vi "Report.vi"() -> ()   [LabVIEW 2019]
uses:
  <vilib>/Utility/NIReport.llb/Report Type.ctl
  <vilib>/addons/_office/excel.llb/Excel Get Data ([str]).vi
  <vilib>/Utility/NIReport.llb/Append Text Table to Report (wrap).vi
  <vilib>/Utility/NIReport.llb/NI_report.lvclass
  <vilib>/Utility/NIReport.llb/NI_ReportGenerationCore.lvlib
  <vilib>/addons/_office/NI_ReportGenerationToolkit.lvlib
  <vilib>/Utility/NIReport.llb/Excel/NI_Excel.lvclass
panel:
  out "data 5":string[][](array[string])
  out "data 4":string[][](array[string])
  out "data 3":string[][](array[string])
  out "data":string[][](array[string])
  out "data 2":string[][](array[string])
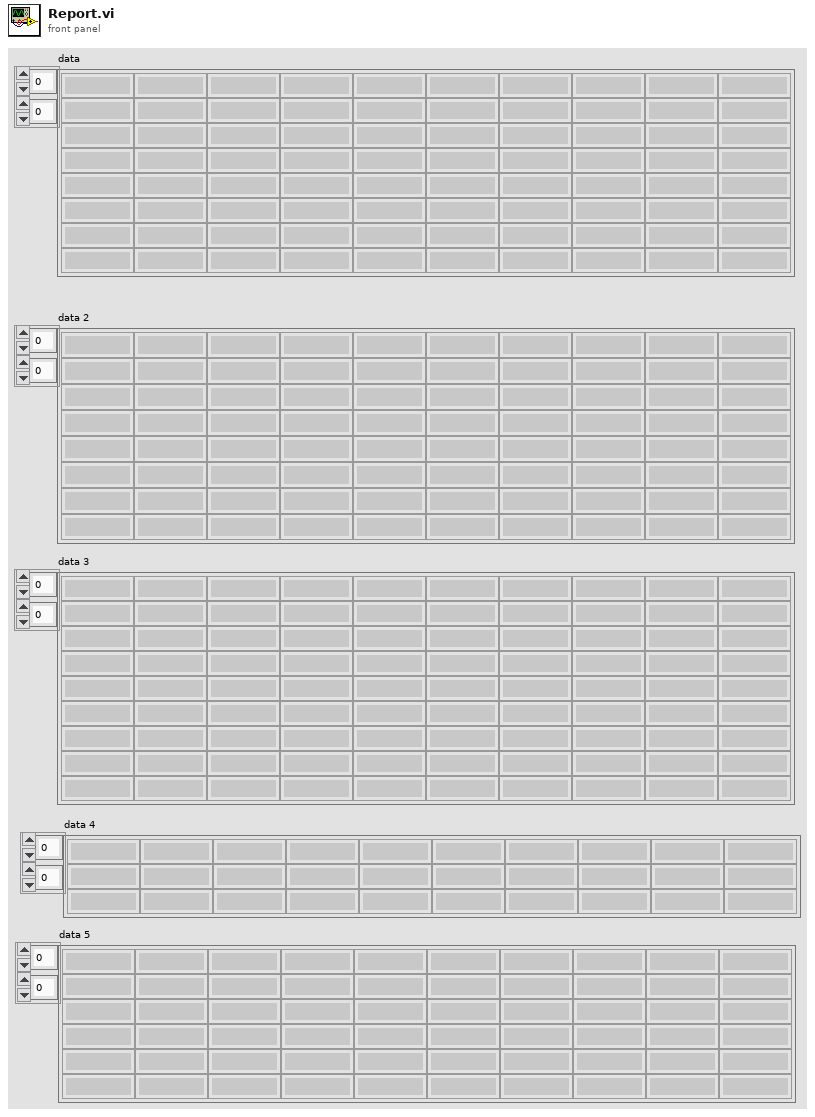
[diagram p1: front panel]
types:
  T1 = typedef "NI_ReportGenerationCore.lvlib/Report Type.ctl" = enum16{"HTML", "Word", "Excel"}
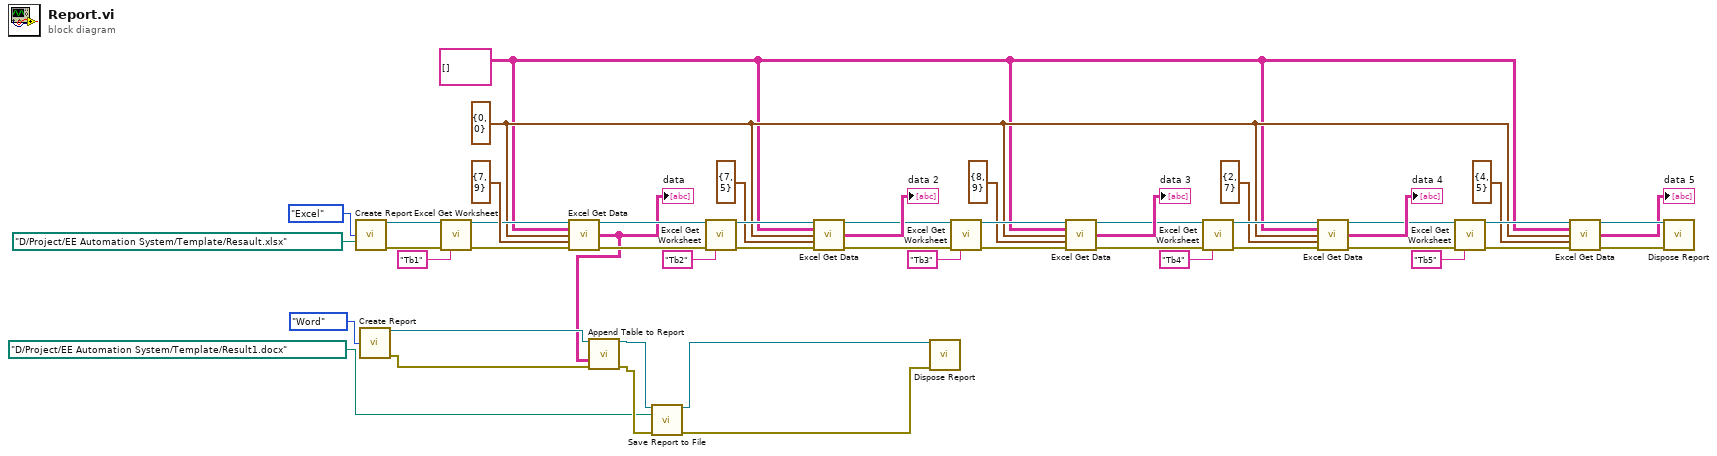
[diagram p0: block diagram]
diagram:
  w7 = string[][] [] ("data type")
  w15 = cluster{"row":i32, "column":i32} {"row"=0, "column"=0} ("start (-1, -1)")
  n1 = call <vilib>:"Create Report.vi"("report type"=Report_Type."Excel", "template (empty)"=path "D:/Project/EE Automation System/Template/Resault.xlsx") -> ("report out"=w43:refnum<class "NI_report.lvclass">, "error out"=w39:errorcluster)  [unwired: 12 in]
  n2 = call <vilib>:"Create Report.vi"("report type"=Report_Type."Word") -> ("report out"=w9:refnum<class "NI_report.lvclass">, "error out"=w8:errorcluster)  [unwired: 13 in]
  n3 = call <vilib>:"Excel Get Worksheet.vi"("report in"=w43, "error in (no error)"=w39, "name (\"\")"="Tb1" ("name (\"\")")) -> ("report out"=w45:refnum<class "NI_report.lvclass">, "error out"=w44:errorcluster)  [unwired: 11 in]
  n4 = call-poly <vilib>:"Excel Get Data.vi"("report in"=w45, "data type"=w7, "start (-1, -1)"=w15, "end (-1, -1)"=cluster{"row":i32, "column":i32} {"row"=7, "column"=9}, "error in (no error)"=w44) -> ("report out"=w36:refnum<class "NI_report.lvclass">, "data"=w1:string[][], "error out"=w35:errorcluster)  [unwired: 8 in]
  "data" <- w1
  n5 = call-poly <vilib>:"Append Table to Report.vi"("report in"=w9, "text data"=w1, "error in (no error)"=w8) -> ("report out"=w6:refnum<class "NI_report.lvclass">, "error out"=w5:errorcluster)  [unwired: 9 in, 2 out]
  n6 = call-dynamic "Save Report to File.vi"("report in"=w6, "report file path"=path "D:/Project/EE Automation System/Template/Result1.docx" ("template (empty)"), "error in (no error)"=w5) -> ("report out"=w3:refnum<class "NI_report.lvclass">, "error out"=w4:errorcluster)  [unwired: 11 in]
  n7 = call <vilib>:"Excel Get Worksheet.vi"("report in"=w36, "error in (no error)"=w35, "name (\"\")"="Tb2" ("name (\"\")")) -> ("report out"=w41:refnum<class "NI_report.lvclass">, "error out"=w40:errorcluster)  [unwired: 11 in]
  n8 = call-poly <vilib>:"Excel Get Data.vi"("report in"=w41, "data type"=w7, "start (-1, -1)"=w15, "end (-1, -1)"=cluster{"row":i32, "column":i32} {"row"=7, "column"=5}, "error in (no error)"=w40) -> ("report out"=w33:refnum<class "NI_report.lvclass">, "data"=→"data 2":string[][], "error out"=w34:errorcluster)  [unwired: 8 in]
  n9 = call-dynamic "Dispose Report.vi"("report in"=w3, "error in (no error)"=w4) -> ()  [unwired: 13 in, 1 out]
  n10 = call <vilib>:"Excel Get Worksheet.vi"("report in"=w33, "error in (no error)"=w34, "name (\"\")"="Tb3" ("name (\"\")")) -> ("report out"=w31:refnum<class "NI_report.lvclass">, "error out"=w30:errorcluster)  [unwired: 11 in]
  n11 = call-poly <vilib>:"Excel Get Data.vi"("report in"=w31, "data type"=w7, "start (-1, -1)"=w15, "end (-1, -1)"=cluster{"row":i32, "column":i32} {"row"=8, "column"=9}, "error in (no error)"=w30) -> ("report out"=w26:refnum<class "NI_report.lvclass">, "data"=→"data 3":string[][], "error out"=w27:errorcluster)  [unwired: 8 in]
  n12 = call <vilib>:"Excel Get Worksheet.vi"("report in"=w26, "error in (no error)"=w27, "name (\"\")"="Tb4" ("name (\"\")")) -> ("report out"=w23:refnum<class "NI_report.lvclass">, "error out"=w24:errorcluster)  [unwired: 11 in]
  n13 = call-poly <vilib>:"Excel Get Data.vi"("report in"=w23, "data type"=w7, "start (-1, -1)"=w15, "end (-1, -1)"=cluster{"row":i32, "column":i32} {"row"=2, "column"=7}, "error in (no error)"=w24) -> ("report out"=w19:refnum<class "NI_report.lvclass">, "data"=→"data 4":string[][], "error out"=w18:errorcluster)  [unwired: 8 in]
  n14 = call <vilib>:"Excel Get Worksheet.vi"("report in"=w19, "error in (no error)"=w18, "name (\"\")"="Tb5" ("name (\"\")")) -> ("report out"=w16:refnum<class "NI_report.lvclass">, "error out"=w17:errorcluster)  [unwired: 11 in]
  n15 = call-poly <vilib>:"Excel Get Data.vi"("report in"=w16, "data type"=w7, "start (-1, -1)"=w15, "end (-1, -1)"=cluster{"row":i32, "column":i32} {"row"=4, "column"=5}, "error in (no error)"=w17) -> ("report out"=w13:refnum<class "NI_report.lvclass">, "data"=→"data 5":string[][], "error out"=w12:errorcluster)  [unwired: 8 in]
  n16 = call-dynamic "Dispose Report.vi"("report in"=w13, "error in (no error)"=w12) -> ()  [unwired: 13 in, 1 out]
